vi "get_concentraion_from_valves.vi"(9 "Mix Cluster":T1={"Ratio"=[0.6, 0.5], "Mix 2"=[12, 12], "Mix 1"=[0, 1]} {"Mix 1" items=["A1"=0, "A2"=1, "A3"=2, "A4"=3, "A5"=12]; "Mix 2" items=["B5"=8, "B6"=9, "B7"=10, "B8"=11, "A5"=12]}, 10 "Valves":u16[](array[ring]) items=["A1", "A2", "A3", "A4", "B1", "B2", "B3", "B4", "B5", "B6", "B7", "B8", "A5"], 11 "Odor Names":string[](array[string])) -> (2 "Mix 2 Odors":string[](array[string]), 3 "Mix 1 Odors":string[](array[string]))   [LabVIEW 2016]
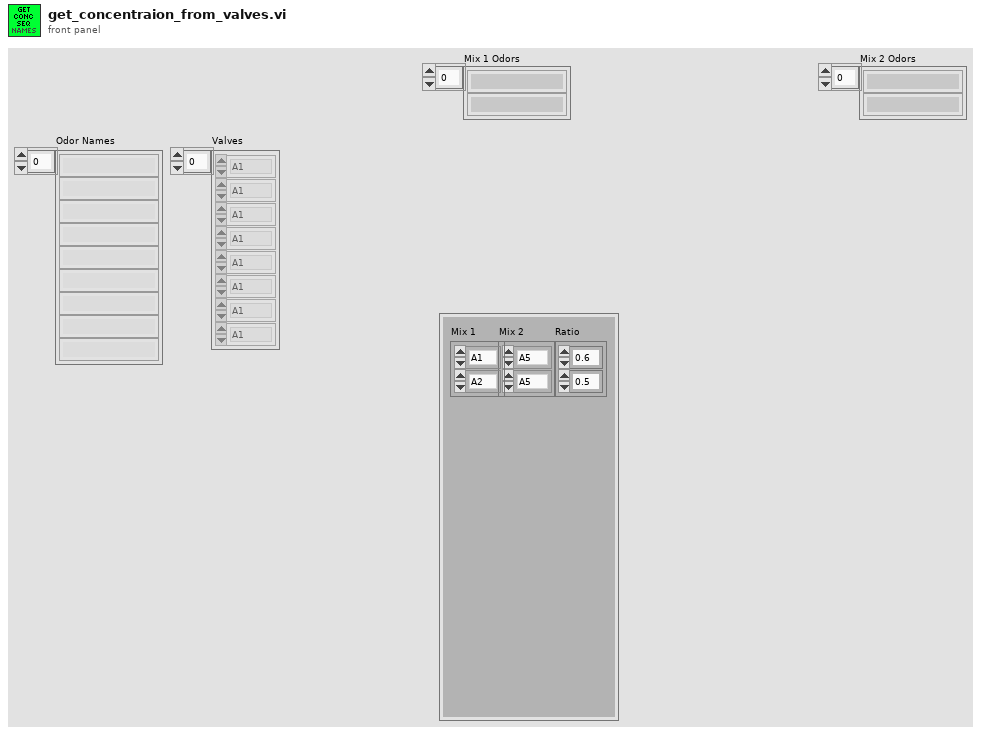
[diagram p1: front panel]
types:
  T1 = cluster{"Ratio":dbl[], "Mix 2":u16[], "Mix 1":u16[]}
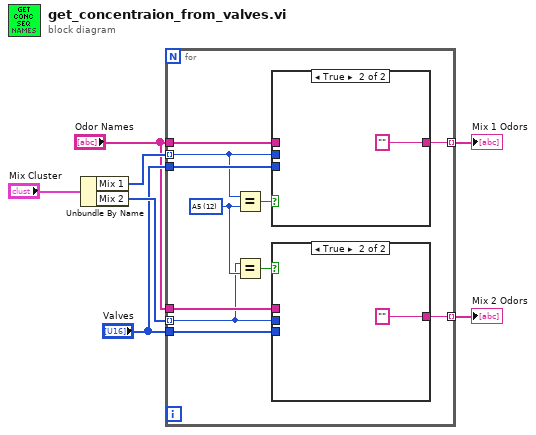
[diagram p0: block diagram]
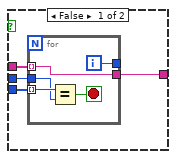
[diagram p2: hidden frame]
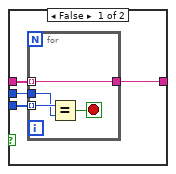
[diagram p3: hidden frame]
diagram:
  n1 = Unbundle By Name("Mix Cluster") -> ("Mix 1"=w6:u16[], "Mix 2"=w5:u16[])
  n2 = for {
    tunnel: "Valves" -> [w18]
    tunnel: w6 -> [w16] mode=indexing
    tunnel: w5 -> [w9] mode=indexing
    tunnel: "Valves" -> [w17]
    tunnel: [w14] -> w1 mode=indexing
    tunnel: "Odor Names" -> [w13]
    tunnel: "Odor Names" -> [w12]
    tunnel: [w11] -> w2 mode=indexing
    w10 = u16 12 items=["A1", "A2", "A3", "A4", "B1", "B2", "B3", "B4", "B5", "B6", "B7", "B8", "A5"] ("Valves")
    n3 = Equal?(x=w16, y=w10) -> (x = y?=w15:bool)
    n4 = Equal?(x=w9, y=w10) -> (x = y?=w8:bool)
    n5 = case shown="True" w15 {
      tunnel: w18 -> [w32 _]
      tunnel: w16 -> [w31 _]
      tunnel: [w29 ""] -> w14
      tunnel: w13 -> [w30 _]
      frame False {
        n6 = for {
          tunnel: w31 -> [w35]
          tunnel: w32 -> [w36] mode=indexing
          tunnel: w30 -> [w33] mode=indexing
          tunnel: [w33] -> w29
          stop <- w34 stop-if-true
          n7 = Equal?(x=w36, y=w35) -> (x = y?=w34:bool)
        }
      }
      frame True {
      }
    }
    n8 = case shown="True" w8 {
      tunnel: w17 -> [w22 _]
      tunnel: w12 -> [w21 _]
      tunnel: [w20 ""] -> w11
      tunnel: w9 -> [w19 _]
      frame False {
        n9 = for {
          tunnel: w19 -> [w26]
          tunnel: w22 -> [w27] mode=indexing
          tunnel: [w24] -> _
          tunnel: w21 -> [w23] mode=indexing
          tunnel: [w23] -> w20
          i -> [w24]
          stop <- w25 stop-if-true
          n10 = Equal?(x=w27, y=w26) -> (x = y?=w25:bool)
        }
      }
      frame True {
      }
    }
  }
  "Mix 2 Odors" <- w2
  "Mix 1 Odors" <- w1
